vi "ShowProgressPercentToArrCtrl.vi"(5 "test time":dbl, 7 "column index":u16, 10 "ref emerg stop btn":refnum<vi>, 11 "ref testcase":refnum<vi>) -> ()   [LabVIEW 2018]
uses:
  Module/Library-Ctrl/Library-Ctrl.lvlib
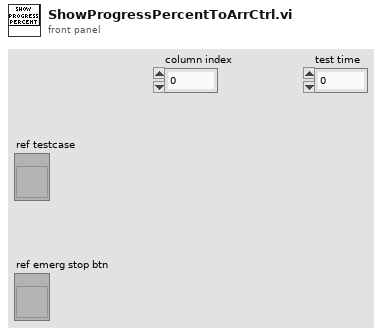
[diagram p1: front panel]
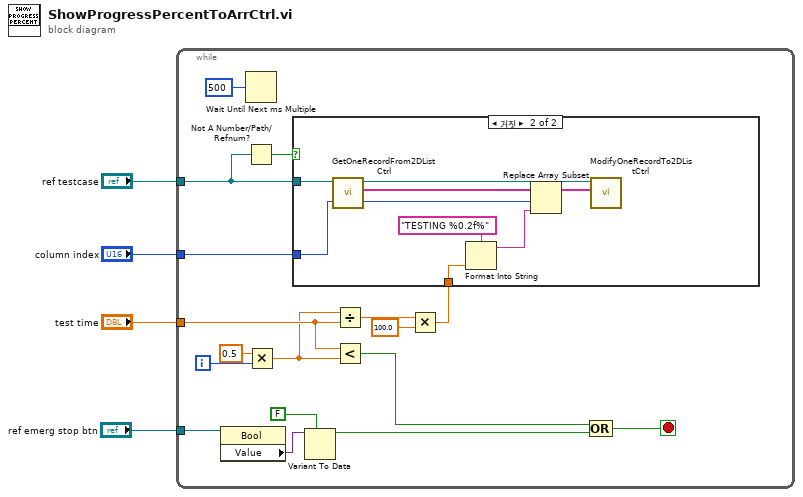
[diagram p0: block diagram]
diagram:
  n1 = while {
    tunnel: "ref testcase" -> [w6]
    tunnel: "column index" -> [w8]
    tunnel: "test time" -> [w18]
    tunnel: "ref emerg stop btn" -> [w13]
    i -> [w21]
    stop <- w10 stop-if-true
    n2 = property class="Bool"(reference=w13) -> ("Value"=w9:variant)  [unwired: 1 in, 2 out]
    n3 = Wait Until Next ms Multiple(millisecond multiple=u32 500 ("대기 시간 (ms)")) -> ()  [unwired: 1 out]
    n4 = Not A Number/Path/Refnum?(number/path/refnum=w6) -> (NaN/Path/Refnum?=w5:bool)
    n5 = Multiply(x=0.5, y=w21) -> (x*y=w17:dbl)
    n6 = Variant To Data(type=FALSE, Variant=w9) -> (data=w11:bool)  [unwired: 1 in, 1 out]
    n7 = Divide(x=w17, y=w18) -> (x/y=w16:dbl)
    n8 = Less?(x=w18, y=w17) -> (x < y?=w12:bool)
    n9 = Multiply(x=w16, y=100.0) -> (x*y=w7:dbl)
    n10 = case shown="거짓" w5 {
      tunnel: w8 -> [_ w22]
      tunnel: w6 -> [_ w29]
      tunnel: w7 -> [_ w25]
      frame True {
      }
      frame False {
        n11 = call "GetOneRecordFrom2DListCtrl.vi"("testcaselist in"=w29) -> ("one record"=w27:string[], "testcaselist out"=w28:refnum<vi>)  [unwired: 9 in]
        n12 = Format Into String(format string="TESTING %0.2f%" ("포맷 문자열"), w25) -> (resulting string=w24:string)  [unwired: 2 in, 1 out]
        n13 = Replace Array Subset(array=w27, new element=w24, index=w22) -> (w23:string[])
        n14 = call "ModifyOneRecordTo2DListCtrl.vi"("arr data"=w23, "multiple list in"=w28) -> ()  [unwired: 9 in, 1 out]
      }
    }
    n15 = Compound Arithmetic op=OR ("복합 연산")(w12, w11) -> (w10:bool)
  }
